vi "LcWebView_Dialog1.vi"() -> ()   [LabVIEW 2018, in "LcWebView.lvclass"]
uses:
  LcWebView.lvclass
  Dialogs/IconType.ctl
  Dialogs/DialogButton.ctl
  Dialogs/ButtonStyles.ctl
  Dialogs/ImageLocation.ctl
  Dialogs/DialogImageInfo.ctl
  Dialogs/DialogInput.ctl
  Dialogs/InputType.ctl
panel:
  in  "Inputs":T1(ring)
  in  "Build In Icon types":T2=enum."Question"
  out "ButtonPressed":string
  in  "Image":T3(ring)
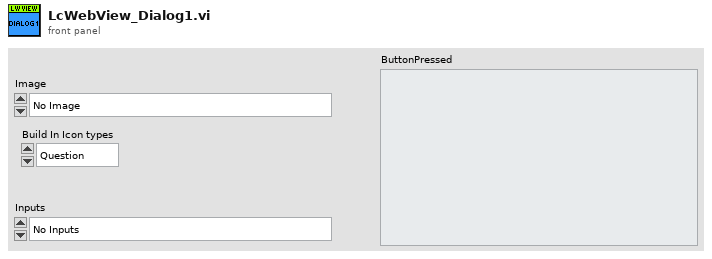
[diagram p1: front panel]
types:
  T1 = enum16{"No Inputs", "One Input", "Many Inputs 1", "Many Inputs 2", "Many Inputs 3", "Many Inputs 4"}
  T2 = typedef "LcWebView.lvclass/IconType.ctl" = enum16{"Sucess", "Error", "Warning", "Info", "Question"}
  T3 = enum16{"No Image", "URL", "Local File", "Image", "Build-In type"}
  T4 = typedef "LcWebView.lvclass/DialogInput.ctl" = cluster{"InputType":T5, "Label":string, "StartValue":variant, "Options":variant, "PlaceholderText":string, "Validation":string}
  T5 = typedef "LcWebView.lvclass/InputType.ctl" = enum16{"Text", "Email", "URL", "Password", "TextArea", "Select", "Radio", "CheckBox", "File", "Range"}
  T6 = typedef "LcWebView.lvclass/ButtonStyles.ctl" = enum16{"Confirm", "Deny", "Cancel"}
  T7 = typedef "LcWebView.lvclass/DialogImageInfo.ctl" = cluster{"Image(URL,Path,Image)":variant, "Width":i32, "Height":i32, "Types":T8}
  T8 = typedef "LcWebView.lvclass/ImageLocation.ctl" = enum16{"Above Title", "Below Title", "Behind Title", "Below Text"}
  T9 = typedef "LcWebView.lvclass/DialogButton.ctl" = cluster{"String":string, "Types":T6, "TextColor":u32, "BgColor":u32}
  T10 = typedef "imagedata.ctl" = cluster{"image type":i32, "image depth":i32, "image":u8[], "mask":u8[], "colors":u32[], "Rectangle":cluster{"left":i16, "top":i16, "right":i16, "bottom":i16}}
  T11 = cluster{"left":i16, "top":i16, "right":i16, "bottom":i16}
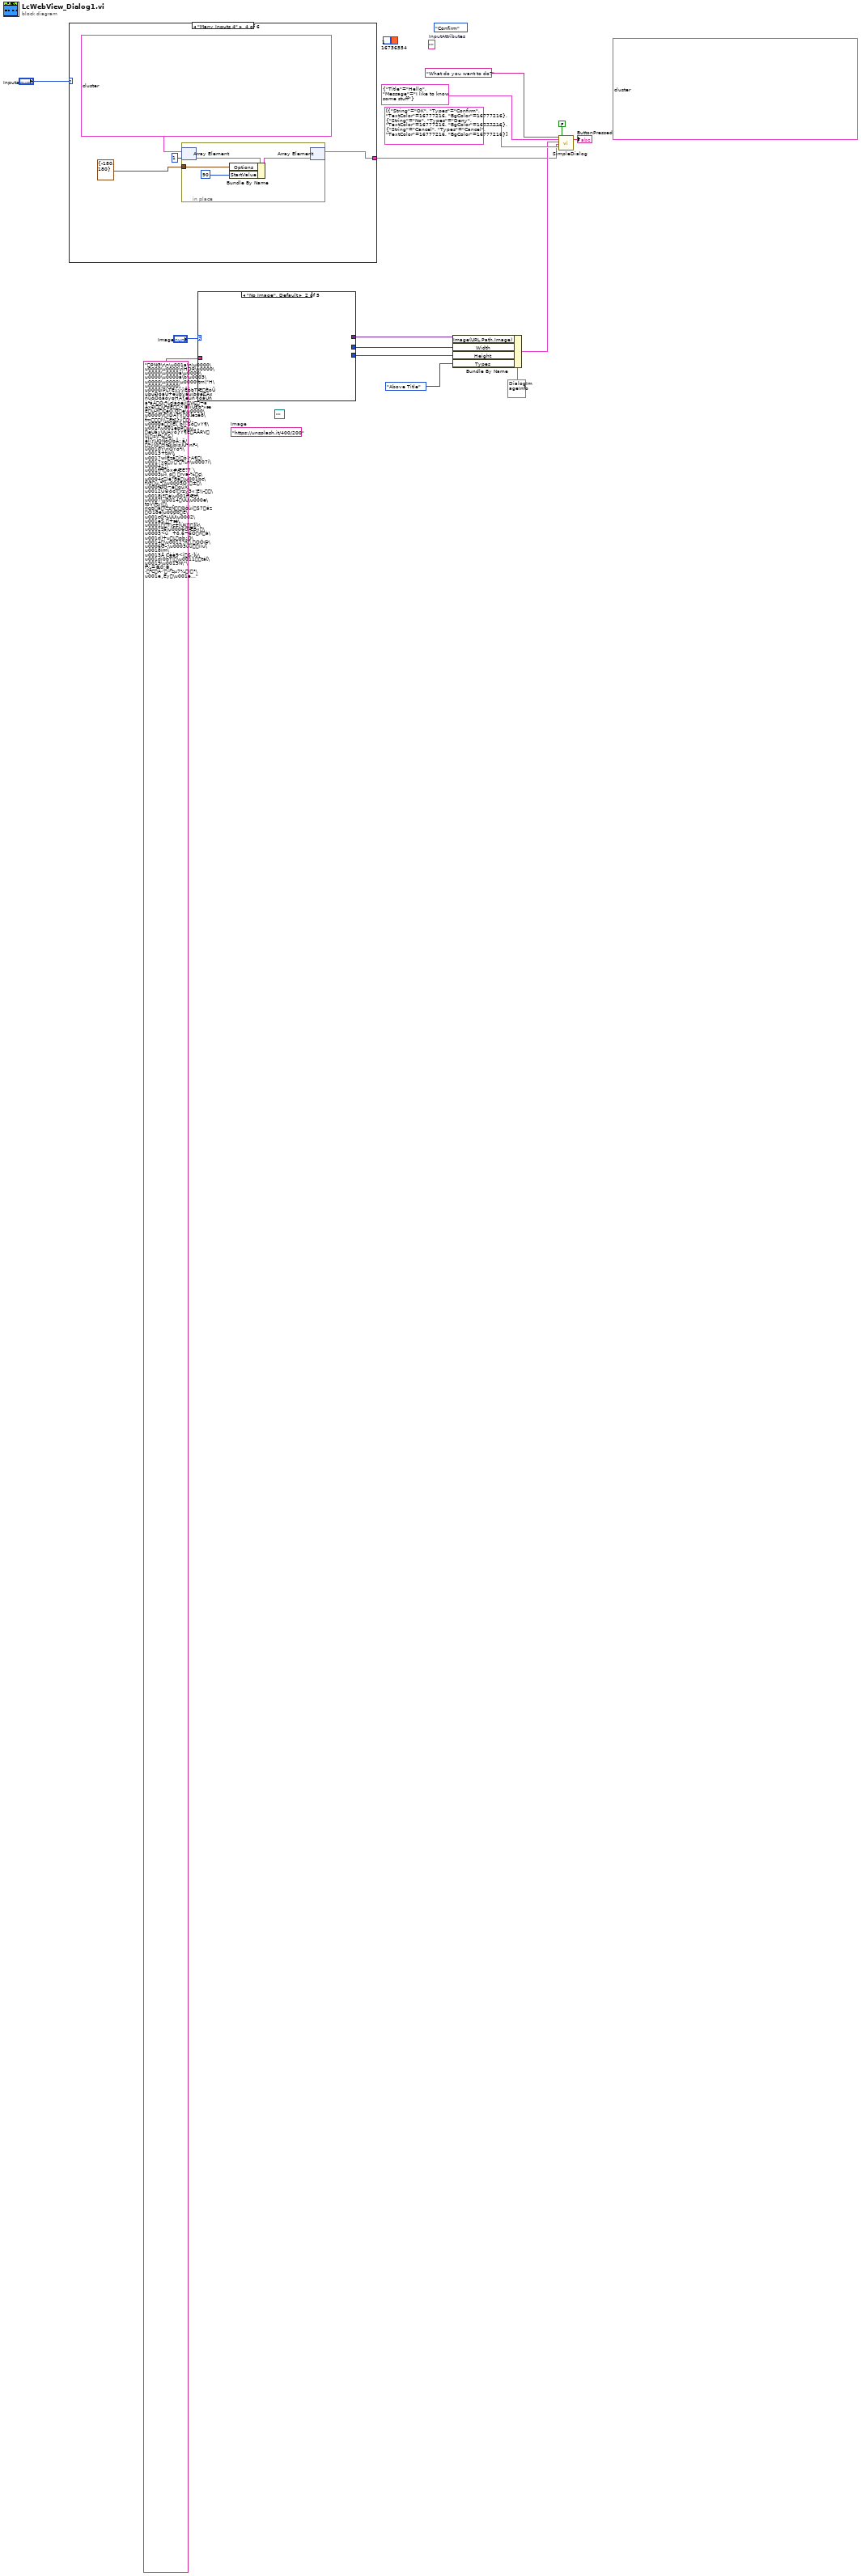
[diagram p0: block diagram]
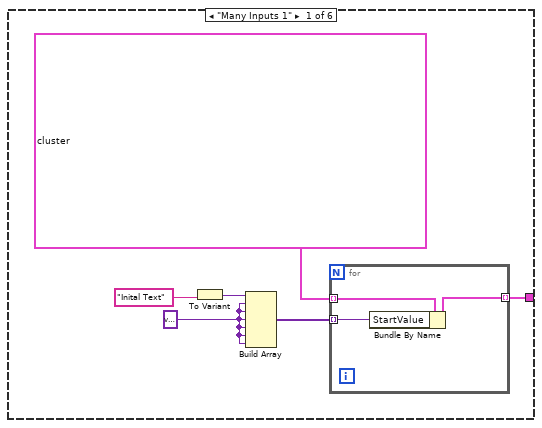
[diagram p2: hidden frame]
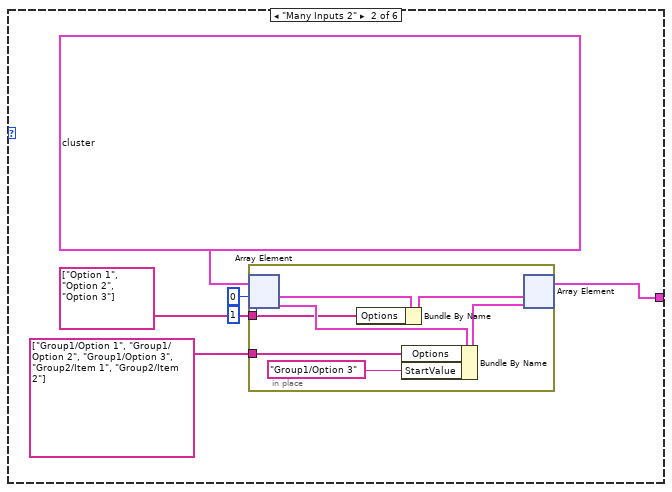
[diagram p3: hidden frame]
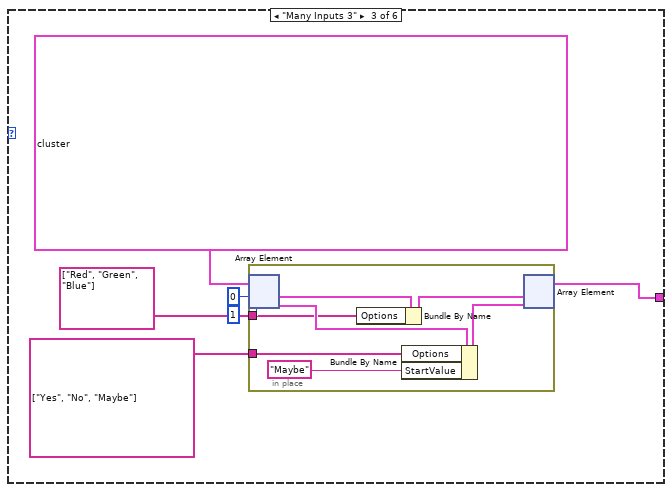
[diagram p4: hidden frame]
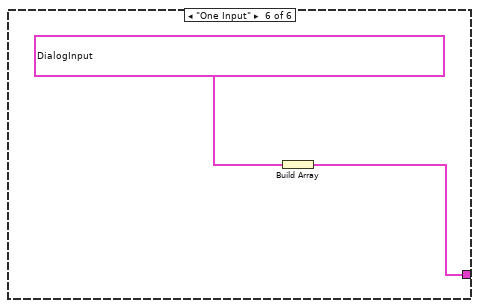
[diagram p6: hidden frame]
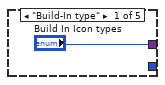
[diagram p7: hidden frame]
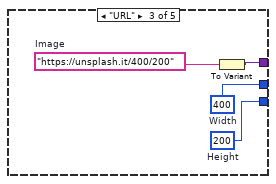
[diagram p8: hidden frame]
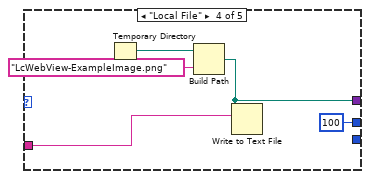
[diagram p9: hidden frame]
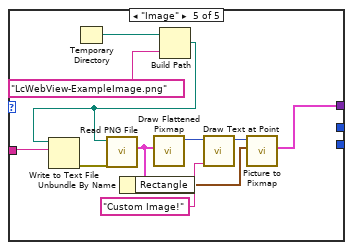
[diagram p10: hidden frame]
diagram:
  (unwired) T4[] [{"InputType"=enum."Select", "Label"="Options", "StartValue"=variant, "Options"=variant, "PlaceholderText"="Selection an Option", "Validation"=""}, {"InputType"=enum."Select", "Label"="Options With Groups", "StartValue"=variant, "Options"=variant, "PlaceholderText"="Select something", "Validation"=""}, {"InputType"=enum."Radio", "Label"="Radio", "StartValue"=variant, "Options"=variant, "PlaceholderText"="", "Validation"=""}, {"InputType"=enum."CheckBox", "Label"="Check?", "StartValue"=variant, "Options"=variant, "PlaceholderText"="", "Validation"=""}, {"InputType"=enum."File", "Label"="File", "StartValue"=variant, "Options"=variant, "PlaceholderText"=" ", "Validation"=""}, {"InputType"=enum."Range", "Label"="Some range", "StartValue"=variant, "Options"=variant, "PlaceholderText"="", "Validation"=""}]
  (unwired) ""  # InputAttributes
  (unwired) u32 16777216 ("TextColor")
  (unwired) u32 16736554 ("BgColor")
  (unwired) ButtonStyles."Confirm" ("Types")
  (unwired) path ""
  (unwired) "https://unsplash.it/400/200"  # Image
  n1 = case shown="\"Many Inputs 4\"" "Inputs" {
    tunnel: [w20 w26 w39 w52 _ w59] -> w1
    frame "Many Inputs 1" {
      w17 = variant
      n2 = To Variant(anything="Inital Text" ("Title")) -> (Variant=w19:variant)
      n3 = Build Array(w19, w17, w17, w17, w17, w17, w17) -> (w16:variant[])
      n4 = for {
        tunnel: T4[] [{"InputType"=enum."Text", "Label"="What's your name", "StartValue"=variant, "Options"=variant, "PlaceholderText"="Text", "Validation"=""}, {"InputType"=enum."Email", "Label"="Email?", "StartValue"=variant, "Options"=variant, "PlaceholderText"="Your email please", "Validation"=""}, {"InputType"=enum."URL", "Label"="Some URL?", "StartValue"=variant, "Options"=variant, "PlaceholderText"="Enter URL here", "Validation"=""}, {"InputType"=enum."Password", "Label"="Pwd", "StartValue"=variant, "Options"=variant, "PlaceholderText"="Your password", "Validation"=""}, {"InputType"=enum."TextArea", "Label"="Some Text", "StartValue"=variant, "Options"=variant, "PlaceholderText"="Text...", "Validation"=""}] -> [w24] mode=indexing
        tunnel: [w23] -> w20 mode=indexing
        tunnel: w16 -> [w22] mode=indexing
        n5 = Bundle By Name(cluster=w24, "StartValue"=w22) -> (w23:T4)
      }
    }
    frame "Many Inputs 2" {
      n6 = in-place {
        in-place-border: string[] ["Group1/Option 1", "Group1/Option 2", "Group1/Option 3", "Group2/Item 1", "Group2/Item 2"] -> [w33]
        in-place-border: string[] ["Option 1", "Option 2", "Option 3"] -> [w32]
        n7 = in-place-array #1(T4[] [{"InputType"=enum."Select", "Label"="Options", "StartValue"=variant, "Options"=variant, "PlaceholderText"="Selection an Option", "Validation"=""}, {"InputType"=enum."Select", "Label"="Options With Groups", "StartValue"=variant, "Options"=variant, "PlaceholderText"="Select something", "Validation"=""}], 0, 1) -> (w37:T4, w35:T4)
        n8 = Bundle By Name(cluster=w37, "Options"=w32) -> (w36:T4)
        n9 = Bundle By Name(cluster=w35, "Options"=w33, "StartValue"="Group1/Option 3" ("Title")) -> (w34:T4)
        n10 = in-place-array #1(w36, w34) -> (w26:T4[])  [unwired: 2 out]
      }
    }
    frame "Many Inputs 3" {
      n11 = in-place {
        in-place-border: string[] ["Yes", "No", "Maybe"] -> [w46]
        in-place-border: string[] ["Red", "Green", "Blue"] -> [w45]
        n12 = in-place-array #2(T4[] [{"InputType"=enum."Radio", "Label"="Radio", "StartValue"=variant, "Options"=variant, "PlaceholderText"="", "Validation"=""}, {"InputType"=enum."Radio", "Label"="Options With Groups", "StartValue"=variant, "Options"=variant, "PlaceholderText"="", "Validation"=""}, {"InputType"=enum."CheckBox", "Label"="Delete?", "StartValue"=variant, "Options"=variant, "PlaceholderText"="Yes", "Validation"=""}], 0, 1) -> (w50:T4, w48:T4)
        n13 = Bundle By Name(cluster=w50, "Options"=w45) -> (w49:T4)
        n14 = Bundle By Name(cluster=w48, "Options"=w46, "StartValue"="Maybe" ("Title")) -> (w47:T4)
        n15 = in-place-array #2(w49, w47) -> (w39:T4[])  [unwired: 2 out]
      }
    }
    frame "Many Inputs 4" {
      n16 = in-place {
        in-place-border: cluster{i32, i32} {-180, 180} -> [w56]
        n17 = in-place-array #3(T4[] [{"InputType"=enum."File", "Label"="File", "StartValue"=variant, "Options"=variant, "PlaceholderText"="", "Validation"=""}, {"InputType"=enum."Range", "Label"="Select a number", "StartValue"=variant, "Options"=variant, "PlaceholderText"="", "Validation"=""}], 1) -> (w58:T4)
        n18 = Bundle By Name(cluster=w58, "Options"=w56, "StartValue"=90) -> (w57:T4)
        n19 = in-place-array #3(w57) -> (w52:T4[])  [unwired: 1 out]
      }
    }
    frame "No Inputs", Default {
    }
    frame "One Input" {
      n20 = Build Array(T4 {"InputType"=enum."Text", "Label"="What's your name", "StartValue"=variant, "Options"=variant, "PlaceholderText"="Text", "Validation"=""} ("DialogInput")) -> (w59:T4[])
    }
  }
  n21 = case shown="\"No Image\", Default" "Image" {
    tunnel: ["Build In Icon types" _ w64 w68 w71] -> w6
    tunnel: [_ _ w63 _ _] -> w5
    tunnel: [_ _ w62 100 ("Width") _] -> w4
    tunnel: "PNG\r\n\u001a\n\u0000\u0000\u0000\rIHDR\u0000\u0000\u0000á\u0000\u0000\u0000á\b\u0003\u0000\u0000\u0000\tm\"H\u0000\u0000\u0000iPLTEÿÿÿËôÞTÆÈóÜùþûÐõáÛ÷èüþýãùíÞøêCÂxñüöÓöãôýøHÃ{éúñ×öåÙñâ²ãÄÓ¡¾çÍâôéjÌVÇ¬áÀxÐÛ³dË×©ÏíÚ£Þ¹»æËÙ­rÏÇêÔ.Qé\u0000\u0000\rIDATxÕ]ézê8\fml\\ZÊt§}ÿ\u0000alË[¨þÌ|·$övY¶\u001f\u001ebPµu_eUåyUUÃÿõ}Ý¶EÁÃRVùj¤\f%&/ëlîYÚQÑöÕbÄ¡ ã/ªÿ[0ºltÐ\bÎ¤)Û¹'nF­\u0010Ý\rÌÕÝó²Î\u0013+tW(\u0017wÌÊzåîò>A¶\u0017xgý¹¾ñ\u0007ï\u00042¿\u001fFfox#ÆE?7´\u0003µ« ø rva­½ç\u0004cZÍê?Bã\u001bc\f|Gù,²\u0005Ô?±\u000fÐÖ~êqüX\u0012Ù®ö¢Ir¥ý3«!E\\­\u0018jºè\u001f³Ætf\u0007\u0014UU\u000e\toV\ftyI\rIqÞã(ª¥ÑØôùí$7ázÔ1ðe\u000bÉ\u001cÒ½ÚÜ\u0002\u001eS.÷æ\u0001Tjç±ÏÙK]ïk\u0002z6\u0006ÖÆB«\u0003<û´ +õ.6¬6Öñà\u001d)+uLpþ¿Ò\u0014\u0012?ñ.OÓ@\u0006G-¡\u0003ûüiÌu\u0018Im\u0013Å Cèè9<î&;]ù\u001dí0bT|\u0011tá[\u0019\u0015N\"\f¾=©0¦©_·³CÃ·'>zµ7¼I°\u001e¸Èy\u001e..." -> [_ _ _ w66 w79]
    frame "Build-In type" {
    }
    frame "No Image", Default {
    }
    frame "URL" {
      w63 = 200  # Height
      w62 = 400  # Width
      w65 = "https://unsplash.it/400/200"  # Image
      n22 = To Variant(anything=w65) -> (Variant=w64:variant)
    }
    frame "Local File" {
      n23 = Temporary Directory() -> (w70:path)
      n24 = Build Path(base path=w70, name or relative path="LcWebView-ExampleImage.png") -> (appended path=w68:path)
      n25 = Write to Text File(file (use dialog)=w68, text=w66) -> ()  [unwired: 2 in, 3 out]
    }
    frame "Image" {
      n26 = Temporary Directory() -> (w81:path)
      n27 = Build Path(base path=w81, name or relative path="LcWebView-ExampleImage.png") -> (appended path=w77:path)
      n28 = Write to Text File(file (use dialog)=w77, text=w79) -> (error out=w78:errorcluster)  [unwired: 2 in, 2 out]
      n29 = call <vilib>:"Read PNG File.vi"("error in (no error)"=w78, "path to PNG file"=w77) -> ("image data"=w73:T10)  [unwired: 7 in, 2 out]
      n30 = Unbundle By Name(w73) -> ("Rectangle"=w72:T11)
      n31 = call <vilib>:"Draw Flattened Pixmap.vi"("image data"=w73) -> ("new picture"=w76:picture)  [unwired: 8 in]
      n32 = call <vilib>:"Draw Text at Point.vi"("text"="Custom Image!", "picture"=w76) -> ("new picture"=w74:picture)  [unwired: 8 in, 1 out]
      n33 = call <vilib>:"Picture to Pixmap.vi"("rect"=w72, "picture"=w74) -> ("image data"=w71:T10)  [unwired: 8 in, 1 out]
    }
  }
  n34 = Bundle By Name(cluster=T7 {"Image(URL,Path,Image)"=variant, "Width"=0, "Height"=0, "Types"=enum."Above Title"} ("DialogImageInfo"), "Image(URL,Path,Image)"=w6, "Width"=w4, "Height"=w5, "Types"=ImageLocation."Above Title") -> (w8:T7)
  n35 = call "SimpleDialog.vi"("Title(If empty Title bar is hidden)"="What do you want to do?", "Message"=cluster{"Title":string, "Message":string} {"Title"="Hello", "Message"="I like to know some stuff"}, "DialogImageInfo"=w8, "Inputs"=w1, "Buttons(OK)"=T9[] [{"String"="OK", "Types"=enum."Confirm", "TextColor"=16777216, "BgColor"=16777216}, {"String"="No", "Types"=enum."Deny", "TextColor"=16777216, "BgColor"=16777216}, {"String"="Cancel", "Types"=enum."Cancel", "TextColor"=16777216, "BgColor"=16777216}], "Closeable?"=FALSE) -> ("ButtonPressed"=→"ButtonPressed":string)  [unwired: 12 in, 1 out]
